vi "Set Attenuation.vi"(8 "error in":errorcluster, 10 "Attenuation":dbl=-100.0, 11 "LTB-1 in":refnum<class "LTB-1.lvclass">) -> (0 "error out":errorcluster, 3 "LTB-1 out":refnum<class "LTB-1.lvclass">)   [LabVIEW 2018, in "LTB-1.lvlib" / "LTB-1.lvclass"]
doc: "This is a dynamically dispatched VI. The child method will use the appropriate protocols to set the attenuation level on the Variable Optical Attenuator. Additionally, the parent method records the set attenuation value.\n\nAuthor: Ron Dexter\nCompany: Luminar\nModified: 5/20/2018"
uses:
  LTB-1.lvclass
  C:/AME Test Engineering/LabVIEW/PPLs/EXFO/Parent/EXFO.lvlibp/EXFO.lvclass
  LTB-1.lvclass/LTB-1.ctl
  PPLs/EXFO/Parent/EXFO.lvlibp/Methods/Read Resource.vi
  3150 Driver/3150.lvlib
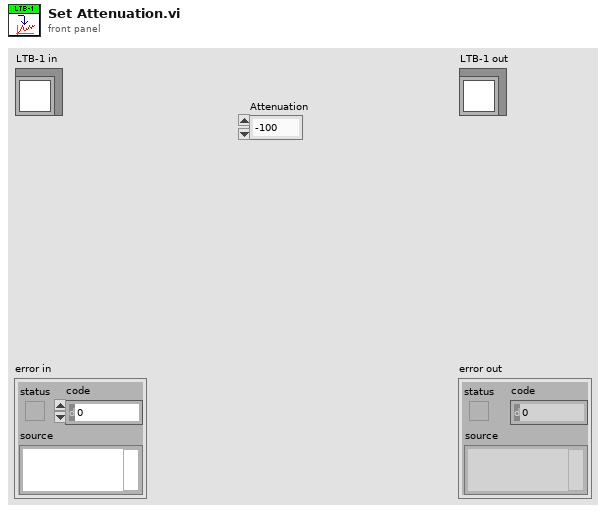
[diagram p1: front panel]
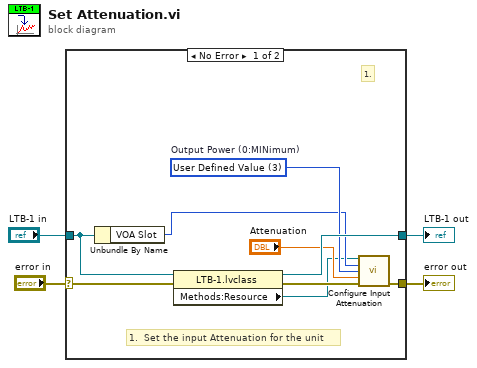
[diagram p0: block diagram]
diagram:
  n1 = case shown="No Error" "error in" {
    selector: "error in" -> [w12 w15]
    tunnel: "LTB-1 in" -> [w11 w14]
    tunnel: [w13 w14] -> w3
    tunnel: [w10 w15] -> w2
    frame No Error {
      w7 = 3 items=["MINimum", "MAXimum", "DEFault", "User Defined Value"]  # Output Power (0:MINimum)
      # "1.  Set the input Attenuation for the unit"
      # "1."
      n2 = Unbundle By Name(w11) -> ("VOA Slot"=w6:i16)
      n3 = property class="LTB-1.lvclass"(reference=w11, error in=w12) -> (reference out=w13:refnum<class "LTB-1.lvclass">, error out=w9:errorcluster, "Methods:Resource"=w5:refnum<visa-resource-name>)
      n4 = call "Configure Input Attenuation.vi"("VISA resource name"=w5, "Platform Slot Number (10)"=w6, "Input Attenuation (0:MINimum)"=w7, "User Defined Attenuation Value (5.0000)"="Attenuation", "error in (no error)"=w9) -> ("error out"=w10:errorcluster)  [unwired: 9 in, 1 out]
    }
    frame Error {
    }
  }
  "error out" <- w2
  "LTB-1 out" <- w3
